vi "math_test.vi"() -> ()   [LabVIEW 2013]
panel:
  out "Magnitude +Math":dbl[][](array[numeric])
  out "Phase + Math":dbl[][](array[numeric])
  out "transposed matrix":dbl[][](array[numeric])
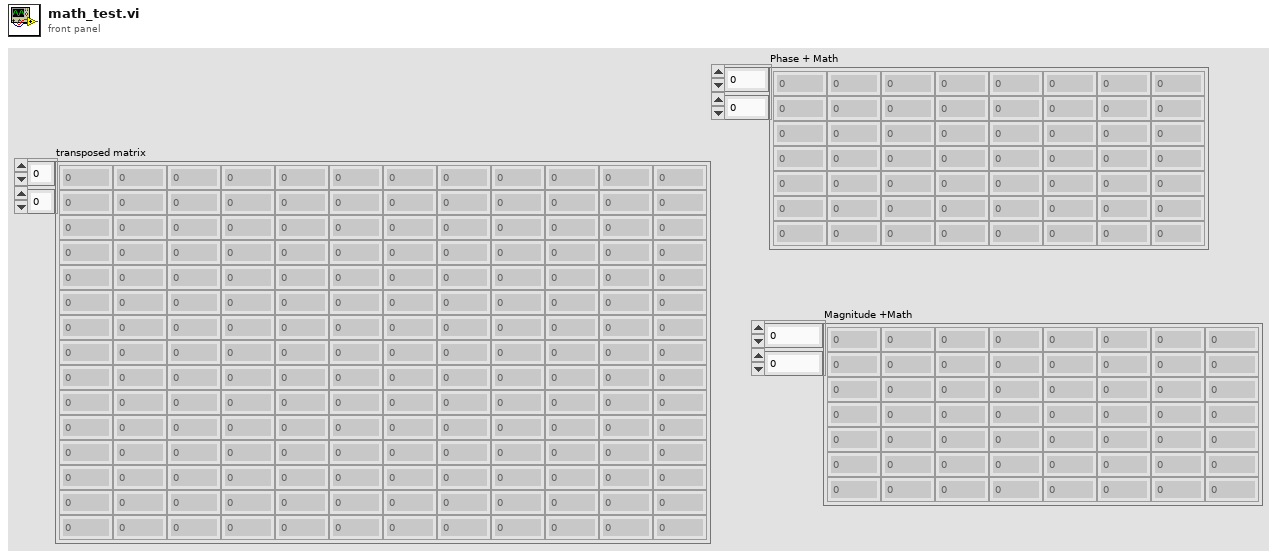
[diagram p1: front panel]
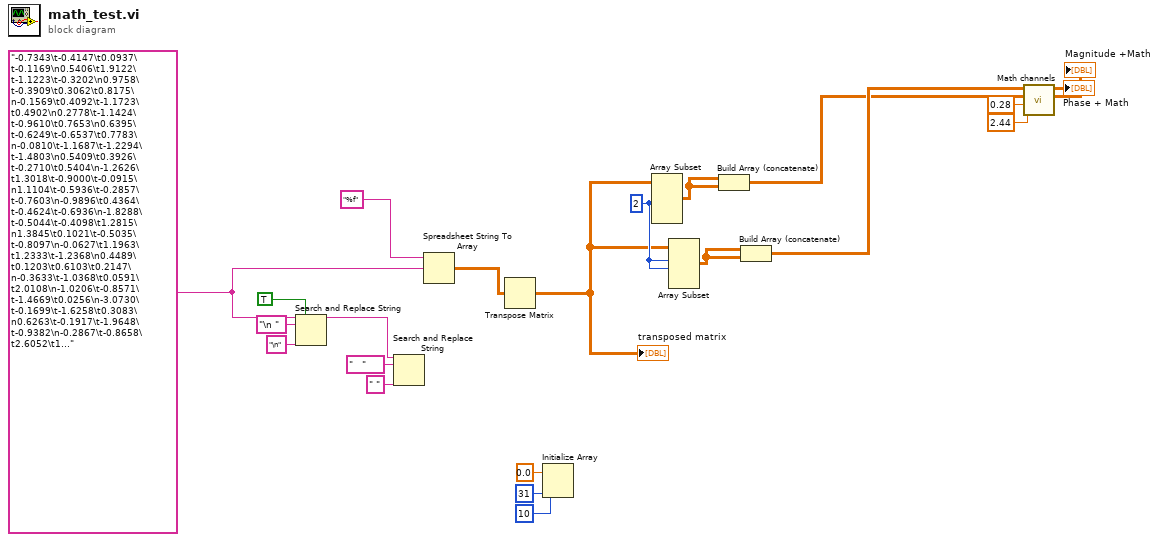
[diagram p0: block diagram]
diagram:
  w13 = 2 ("length")
  w14 = "-0.7343\t-0.4147\t0.0937\t-0.1169\n0.5406\t1.9122\t-1.1223\t-0.3202\n0.9758\t-0.3909\t0.3062\t0.8175\n-0.1569\t0.4092\t-1.1723\t0.4902\n0.2778\t-1.1424\t-0.9610\t0.7653\n0.6395\t-0.6249\t-0.6537\t0.7783\n-0.0810\t-1.1687\t-1.2294\t-1.4803\n0.5409\t0.3926\t-0.2710\t0.5404\n-1.2626\t1.3018\t-0.9000\t-0.0915\n1.1104\t-0.5936\t-0.2857\t-0.7603\n-0.9896\t0.4364\t-0.4624\t-0.6936\n-1.8288\t-0.5044\t-0.4098\t1.2815\n1.3845\t0.1021\t-0.5035\t-0.8097\n-0.0627\t1.1963\t1.2333\t-1.2368\n0.4489\t0.1203\t0.6103\t0.2147\n-0.3633\t-1.0368\t0.0591\t2.0108\n-1.0206\t-0.8571\t-1.4669\t0.0256\n-3.0730\t-0.1699\t-1.6258\t0.3083\n0.6263\t-0.1917\t-1.9648\t-0.9382\n-0.2867\t-0.8658\t2.6052\t1.6742\n-0.1973\t0.1807\t0.9724\t0.1250\n0.4056\t1.2665\t0.2570\t0.5301\n-1.4193\t-0.2512\t-0.9742\t-0.9521\n-0.7294\t-0.2046\t-1.1464\t0.8540\n1.1473\t-2.2015\t0.5476\t0.3891\n0.5979\t-0.7745\t1.5651\t-1.1560\n-1.2813\t-1.3933\t-1.6933\t0.0397\n-2.2033\t-0.3862\t-0.4494\t-0.4506\n-0.5712\t0.5256\t-0.0843\t0.1092\n0.2140\t1.5233\t-1.9920\t-0.2506\n0.9424\t1.7985\t0.8412\t-0.1899\n"
  n1 = Search and Replace String(replace all?=TRUE ("replace all? (F)"), input string=w14, search string="\n ", replace string="\n" ("replace string (\"\")")) -> (result string=w16:string)  [unwired: 4 in, 3 out]
  n2 = Search and Replace String(input string=w16, search string="   ", replace string=" " ("replace string (\"\")")) -> ()  [unwired: 5 in, 4 out]
  n3 = Spreadsheet String To Array(format string="%f", spreadsheet string=w14) -> (array=w21:dbl[][])  [unwired: 2 in]
  n4 = Transpose Matrix(1:w21) -> (0:w12:dbl[][])
  "transposed matrix" <- w12
  n5 = Initialize Array(0.0 ("element"), 10 ("dimension size"), 31 ("dimension size")) -> ()  [unwired: 1 out]
  n6 = Array Subset(array=w12, length (row)=w13) -> (w8:dbl[][])  [unwired: 3 in]
  n7 = Array Subset(array=w12, index (row)=w13, length (row)=w13) -> (w7:dbl[][])  [unwired: 2 in]
  n8 = Build Array (concatenate)(w8, w8) -> (w5:dbl[][])
  n9 = Build Array (concatenate)(w7, w7) -> (w6:dbl[][])
  n10 = call "Math channels.vi"("b"=2.44, "a"=0.28, "Magnitude"=w5, "Phase"=w6) -> ("Magnitude +Math"=→"Magnitude +Math":dbl[][], "Phase + Math"=→"Phase + Math":dbl[][])  [unwired: 6 in]
